vi "Lab 9 Exercise 5 - Temperature Logger.vi"() -> ()   [LabVIEW 2023]
uses:
  <vilib>/Analysis/baseanly.llb/Mean (DBL).vi
  <vilib>/Analysis/NI_AALBase.lvlib
panel:
  out "Mean":dbl
  out "Min Value":dbl
  out "Max Value":dbl
  out "#Index":i32
  in  "?":bool
  out "Current Data":dbl(slide) scale=0.0..100.0
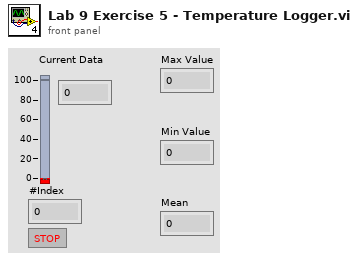
[diagram p1: front panel]
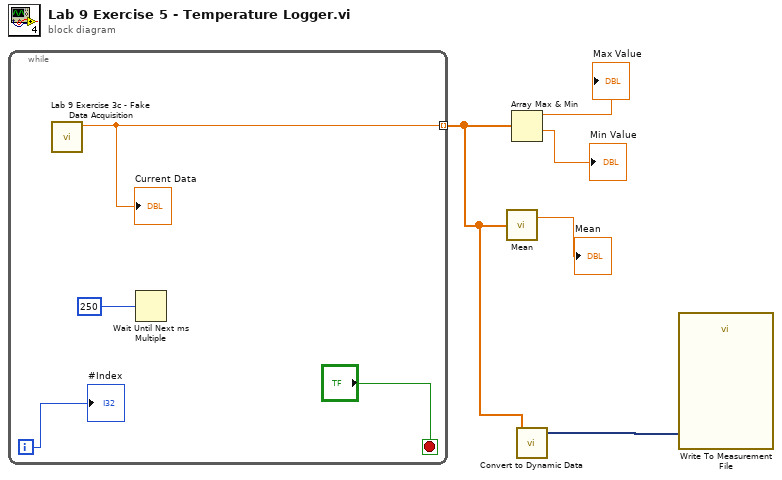
[diagram p0: block diagram]
diagram:
  n1 = while {
    tunnel: [w8] -> w2 mode=indexing
    i -> [w9]
    stop <- "?" stop-if-true
    n2 = call "Lab 9 Exercise 3c - Fake Data Acquisition.vi"() -> ("Temperature"=w8:dbl)  [unwired: 11 in]
    "Current Data" <- w8
    n3 = Wait Until Next ms Multiple(millisecond multiple=250) -> ()  [unwired: 1 out]
    "#Index" <- w9
  }
  n4 = call-poly <vilib>:"Mean.vi"("X"=w2) -> ("mean"=→"Mean":dbl)  [unwired: 1 out]
  n5 = Array Max & Min(array=w2) -> (max value=→"Max Value":dbl, min value=→"Min Value":dbl)  [unwired: 2 out]
  n6 = call "Convert to Dynamic Data"("Array"=w2) -> ("Dynamic Data Type"=w1:dynamicdata)  [unwired: 3 in]
  n7 = call "Write To Measurement File"("Signals"=w1) -> ()  [unwired: 16 in, 3 out]
